vi "Open Front Panel.vi"(7 "Activate?":bool, 8 "error in (no error)":errorcluster, 9 "Front Panel Window:State":T1(ring), 10 "View Hierarchy Level":i32, 11 "GUI View Actor in":refnum<class "GUI View Actor.lvclass">) -> (0 "error out":errorcluster, 3 "GUI View Actor out":refnum<class "GUI View Actor.lvclass">)   [LabVIEW 2017, in "GUI Views.lvlib" / "GUI View Actor.lvclass"]
doc: "Opens the Front Panel of a specified Actor Core VI of the the specified View class hierarchy. The method is active only if the GUI View is not contained. The Front Panel is specified by: \n\n<b> View Hierarchy Level</b> the level on the subclassing hierarchy of the GUI View actor, it is used to choose the Actor Core Front Panel among all the exisiting sublcasses of the GUI VIew Actor present in the View specified above"
uses:
  GUI View Actor.lvclass
  GUI View Actor.lvclass/GUI View Actor.ctl
  properties/Read Managed by Container.vi
  <vilib>/ActorFramework/Message Enqueuer/Equals Not A Refnum.vi
  <vilib>/ActorFramework/Message Enqueuer/Message Enqueuer.lvclass
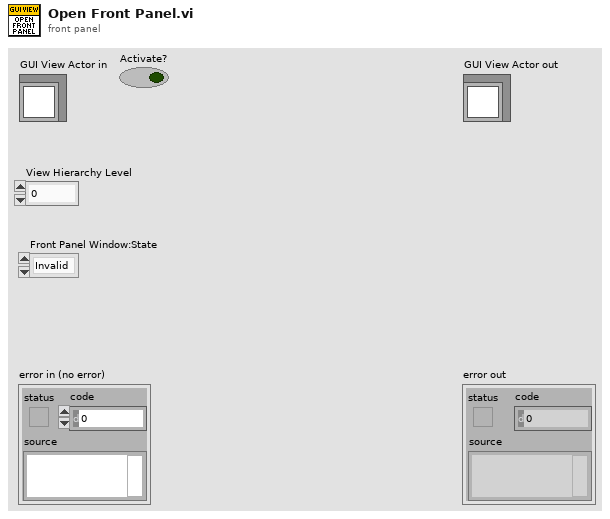
[diagram p1: front panel]
types:
  T1 = enum32{"Invalid", "Standard", "Closed", "Hidden", "Minimized", "Maximized"}
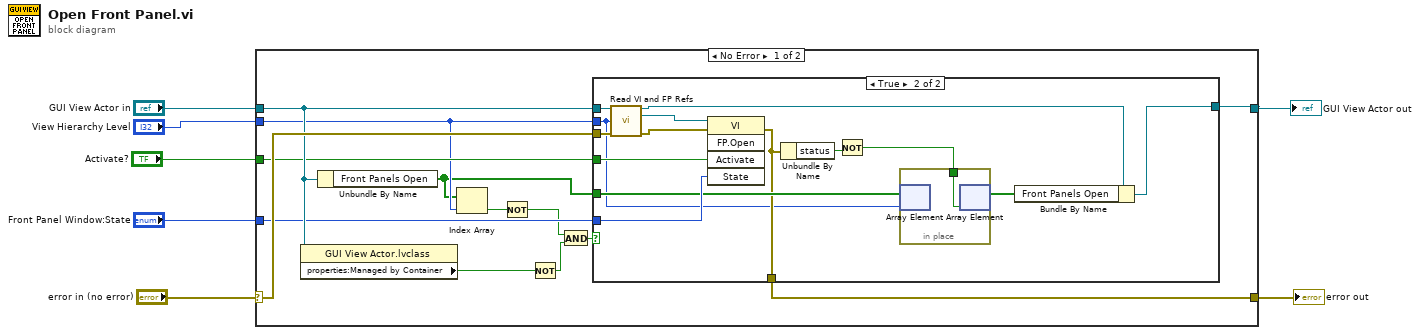
[diagram p0: block diagram]
diagram:
  n1 = case shown="No Error" "error in (no error)" {
    selector: "error in (no error)" -> [w20 w39]
    tunnel: [w18 w39] -> w6
    tunnel: [w19 w38] -> w4
    tunnel: "GUI View Actor in" -> [w16 w38]
    tunnel: "Front Panel Window:State" -> [w15 _]
    tunnel: "View Hierarchy Level" -> [w9 _]
    tunnel: "Activate?" -> [w10 _]
    frame No Error {
      n2 = property class="GUI View Actor.lvclass"(reference=w16) -> ("properties:Managed by Container"=w17:bool)  [unwired: 1 in, 2 out]
      n3 = Unbundle By Name(w16) -> ("Front Panels Open"=w8:bool[])
      n4 = Index Array(array=w8, index=w9) -> (element=w14:bool)
      n5 = Not(x=w14) -> (.not. x?=w12:bool)
      n6 = Not(x=w17) -> (.not. x?=w13:bool)
      n7 = And(x=w12, y=w13) -> (x .and. y?=w11:bool)
      n8 = case shown="True" w11 {
        tunnel: w15 -> [_ w31]
        tunnel: w20 -> [w21 w35]
        tunnel: w9 -> [_ w23]
        tunnel: [w22 w25] -> w19
        tunnel: [w21 w28] -> w18
        tunnel: w16 -> [w22 w32]
        tunnel: w10 -> [_ w30]
        tunnel: w8 -> [_ w29]
        frame False {
        }
        frame True {
          n9 = call "Read VI and FP Refs.vi"("GUI View Actor in"=w32, "View Hierarchy Level"=w23, "error in (no error)"=w35) -> ("GUI View Actor out"=w33:refnum<class "GUI View Actor.lvclass">, "VI Ref"=w36:refnum<vi>, "error out"=w34:errorcluster)  [unwired: 8 in, 2 out]
          n10 = invoke class="VI" method="FP.Open"(reference=w36, error in=w34, "Activate"=w30, "State"=w31) -> (error out=w28:errorcluster)  [unwired: 1 in, 4 out]
          n11 = Unbundle By Name(w28) -> ("status"=w27:bool)
          n12 = Not(x=w27) -> (.not. x?=w26:bool)
          n13 = in-place {
            in-place-border: w26 -> [w37]
            n14 = in-place-array #1(w29, w23) -> ()  [unwired: 1 out]
            n15 = in-place-array #1(w37) -> (w24:bool[])  [unwired: 1 out]
          }
          n16 = Bundle By Name(cluster=w33, "Front Panels Open"=w24) -> (w25:refnum<class "GUI View Actor.lvclass">)
        }
      }
    }
    frame Error {
    }
  }
  "error out" <- w6
  "GUI View Actor out" <- w4
